vi "ParseTree_Reparent_Child.vi"(8 "index of child in new parent":i32, 9 "child":i32, 10 "new parent":i32, 11 "Parse Tree in":T1[](array[typedef])) -> (3 "Parse Tree out":T1[](array[typedef]))   [LabVIEW 2021]
uses:
  <resource>/MathScriptParser/Statement.ctl
  <resource>/MathScriptParser/NodeType.ctl
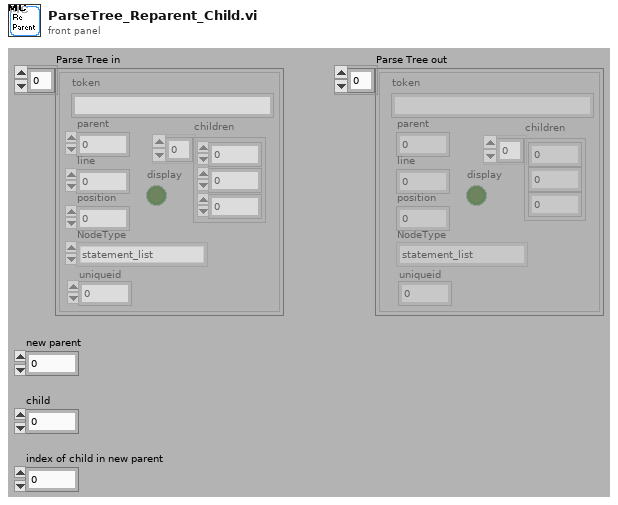
[diagram p1: front panel]
types:
  T1 = typedef "Statement.ctl" = cluster{"parent":u32, "children":u32[], "token":string, "NodeType":T2, "line":u32, "display":bool, "position":u32, "uniqueid":u32}
  T2 = typedef "NodeType.ctl" = enum16{"statement_list", "expression_list", "matrix", "row", "command", "function_1_1", "function_1_N", "function_N_1", "function_N_N", "operator", "assignment", "for", "if", "switch", "while", "try", "range", "identifier", "struct_field", "constant", "udfunction_1_1", "udfunction_1_N", "udfunction_N_1", "udfunction_N_N", "udfunction_0_0", "udfunction_0_1", "udfunction_0_N", "udfunction_1_0", "udfunction_N_0", "function_0_1", "function_0_N", "struct_ref", "array_ref", "cell_array_ref", "cell_matrix"}
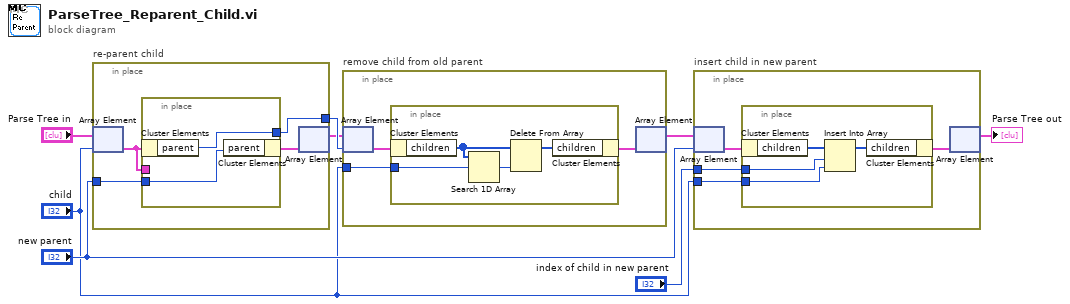
[diagram p0: block diagram]
diagram:
  n1 = in-place "re-parent child" {
    in-place-border: "new parent" -> [w12]
    in-place-border: [w11] -> w7
    n2 = in-place-array #1("Parse Tree in", "child") -> (w10:T1)
    n3 = in-place {
      in-place-border: w12 -> [w13]
      in-place-border: w10 -> [_]
      in-place-border: [w14] -> w11
      n4 = in-place-cluster #2(w10) -> ("parent"=w14:u32)
      n5 = in-place-cluster #2("parent"=w13) -> (w9:T1)
    }
    n6 = in-place-array #1(w9) -> (w6:T1[])  [unwired: 1 out]
  }
  n7 = in-place "remove child from old parent" {
    in-place-border: "child" -> [w17]
    n8 = in-place-array #3(w6, w7) -> (w16:T1)
    n9 = in-place {
      in-place-border: w17 -> [w21]
      n10 = in-place-cluster #4(w16) -> ("children"=w19:u32[])
      n11 = Search 1D Array(1D array=w19, element=w21) -> (index of element=w20:i32)  [unwired: 1 out]
      n12 = Delete From Array(array=w19, index=w20) -> (array with subset deleted=w18:u32[])  [unwired: 1 in, 1 out]
      n13 = in-place-cluster #4("children"=w18) -> (w15:T1)
    }
    n14 = in-place-array #3(w15) -> (w5:T1[])  [unwired: 1 out]
  }
  n15 = in-place "insert child in new parent" {
    in-place-border: "index of child in new parent" -> [w25]
    in-place-border: "child" -> [w24]
    n16 = in-place-array #5(w5, "new parent") -> (w23:T1)
    n17 = in-place {
      in-place-border: w25 -> [w29]
      in-place-border: w24 -> [w28]
      n18 = in-place-cluster #6(w23) -> ("children"=w27:u32[])
      n19 = Insert Into Array(array=w27, index=w29, new element=w28) -> (w26:u32[])
      n20 = in-place-cluster #6("children"=w26) -> (w22:T1)
    }
    n21 = in-place-array #5(w22) -> (→"Parse Tree out":T1[])  [unwired: 1 out]
  }
